vi "Subscribe (Array).vi"(6 "timeout (1000ms)":i32=1000, 8 "error in (no error)":errorcluster, 10 "Topic Subscriptions":T3[](array[typedef]), 11 "Client in":refnum<class "Client.lvclass">) -> (0 "error out":errorcluster, 2 "Subscription Success":T1[](array[typedef]), 3 "Client out":refnum<class "Client.lvclass">)   [LabVIEW 2013, in "MQTT Client.lvlib" / "Client.lvclass"]
uses:
  Client.lvclass
  <vilib>/LabVIEW Open Source Project/MQTT Control Packets/Control Packets/SUBSCRIBE/Topic Subscription -- cluster.ctl
  <vilib>/LabVIEW Open Source Project/MQTT Control Packets/Control Packets/ControlPacket/QualityOfService -- enum.ctl
  <vilib>/LabVIEW Open Source Project/MQTT Control Packets/Control Packets/SUBACK/Subscription Success Code.ctl
  <vilib>/LabVIEW Open Source Project/MQTT Connection/MQTT_Base/Base Class/MQTT_Base.lvclass
  <vilib>/LabVIEW Open Source Project/MQTT Control Packets/Control Packets/ControlPacket/ControlPacket.lvclass
  <vilib>/LabVIEW Open Source Project/MQTT Control Packets/Control Packets/SUBSCRIBE/SUBSCRIBE.lvclass
  <vilib>/LabVIEW Open Source Project/MQTT Control Packets/Control Packets/SUBACK/SUBACK.lvclass
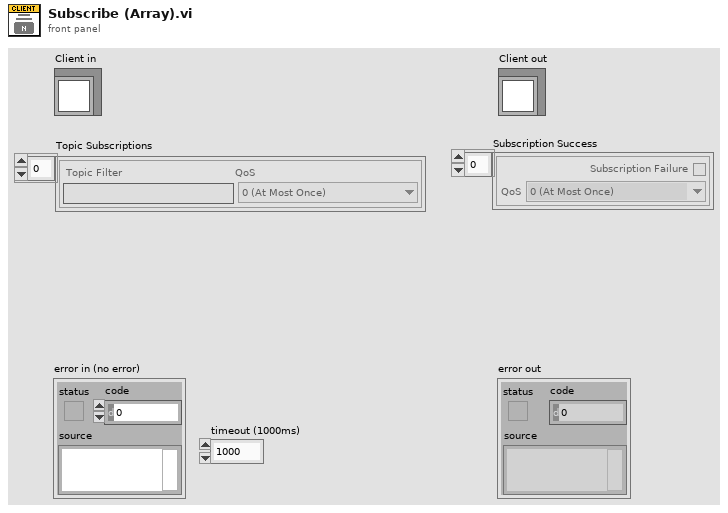
[diagram p1: front panel]
types:
  T1 = typedef "MQTT_Control_Packets.lvlib/SUBACK.lvclass/Subscription Success Code.ctl" = cluster{"Subscription Failure":bool, "QoS":T2}
  T2 = typedef "MQTT_Control_Packets.lvlib/ControlPacket.lvclass/QualityOfService -- enum.ctl" = enum16{"0 (At Most Once)", "1 (At Least Once)", "2 (Exactly Once)"}
  T3 = typedef "MQTT_Control_Packets.lvlib/SUBSCRIBE.lvclass/Topic Subscription -- cluster.ctl" = cluster{"Topic Filter":string, "QoS":T2}
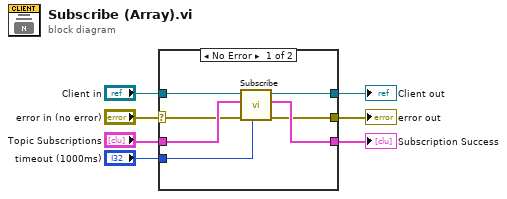
[diagram p0: block diagram]
diagram:
  n1 = case shown="No Error" "error in (no error)" {
    selector: "error in (no error)" -> [w9 w16]
    tunnel: [w10 w16] -> w6
    tunnel: [w13 w15] -> w4
    tunnel: "Client in" -> [w14 w15]
    tunnel: [w11 _] -> w3
    tunnel: "Topic Subscriptions" -> [w12 _]
    tunnel: "timeout (1000ms)" -> [w8 _]
    frame No Error {
      n2 = call <vilib>:"Subscribe.vi"("timeout (1000 ms)"=w8, "error in (no error)"=w9, "Topic Subscriptions"=w12, "MQTT_Base in"=w14) -> ("error out"=w10:errorcluster, "Subscription Success"=w11:T1[], "MQTT_Base out"=w13:refnum<class "Client.lvclass">)  [unwired: 4 in, 1 out]
    }
    frame Error {
    }
  }
  "error out" <- w6
  "Client out" <- w4
  "Subscription Success" <- w3
